vi "Draw Color Band.vi"(8 "error in (no error)":errorcluster, 9 "Range":dbl, 10 "Ideal":dbl, 11 "GaugeIndicator in":refnum<class "GaugeIndicator.lvclass">) -> (0 "error out":errorcluster, 2 "Color Band":picture, 3 "GaugeIndicator out":refnum<class "GaugeIndicator.lvclass">)   [LabVIEW 2020, in "VolatusGUIElements.lvlib" / "GaugeIndicator.lvclass"]
uses:
  GaugeIndicator.lvclass
  GaugeIndicator.lvclass/GaugeIndicator.ctl
panel:
  in  "Gauge":dbl(knob)=1600.0 scale=0.0..2500.0
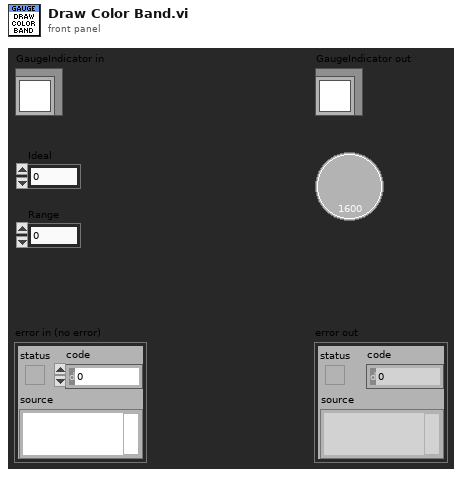
[diagram p1: front panel]
types:
  T1 = cluster{"Width":u16, "Style":enum32{"Solid", "Dash", "Dot", "DashDot", "DashDotDot"}}
  T2 = cluster{"left":i16, "top":i16, "right":i16, "bottom":i16}
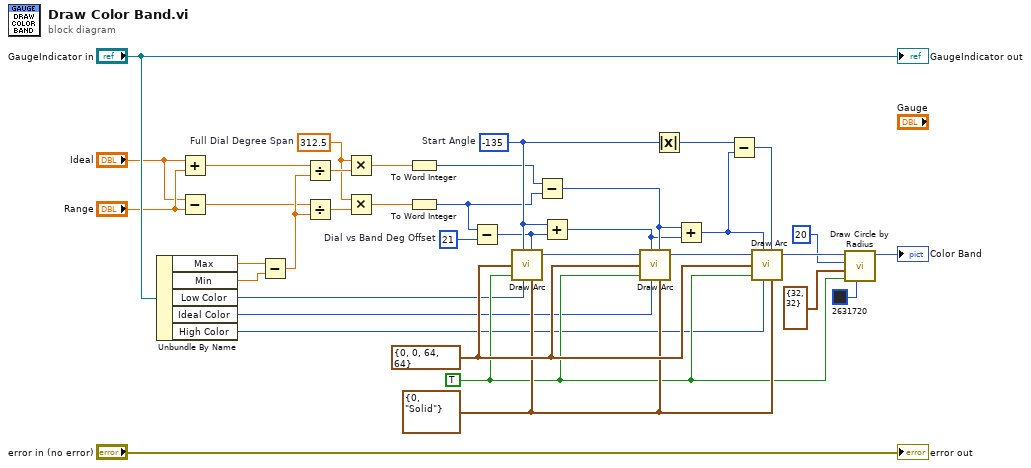
[diagram p0: block diagram]
diagram:
  w7 = i16 21  # Dial vs Band Deg Offset
  w14 = 312.5  # Full Dial Degree Span
  w10 = i16 -135  # Start Angle
  w34 = T1 {"Width"=0, "Style"=enum."Solid"} ("pen")
  w29 = TRUE ("fill?(F)")
  w35 = T2 {"left"=0, "top"=0, "right"=64, "bottom"=64} ("rect")
  n1 = Unbundle By Name("GaugeIndicator in") -> ("Max"=w22:dbl, "Min"=w21:dbl, "Low Color"=w25:u32, "Ideal Color"=w24:u32, "High Color"=w23:u32)
  n2 = Add(x="Ideal", y="Range") -> (x+y=w12:dbl)
  n3 = Subtract(x="Ideal", y="Range") -> (x-y=w8:dbl)
  n4 = Subtract(x=w22, y=w21) -> (x-y=w15:dbl)
  n5 = Divide(x=w12, y=w15) -> (x/y=w19:dbl)
  n6 = Divide(x=w8, y=w15) -> (x/y=w18:dbl)
  n7 = Multiply(x=w14, y=w19) -> (x*y=w11:dbl)
  n8 = Multiply(x=w14, y=w18) -> (x*y=w13:dbl)
  n9 = To Word Integer(number=w11) -> (16bit integer=w6:i16)
  n10 = To Word Integer(number=w13) -> (16bit integer=w3:i16)
  n11 = Subtract(x=w3, y=w7) -> (x-y=w2:i16)
  n12 = call <vilib>:"Draw Arc.vi"("start angle[degrees]"=w10, "rect"=w35, "fill?(F)"=w29, "color(black)"=w25, "arc size[degrees]"=w2, "pen"=w34) -> ("new picture"=w36:picture)  [unwired: 3 in]
  n13 = Subtract(x=w6, y=w3) -> (x-y=w5:i16)
  n14 = Add(x=w10, y=w2) -> (x+y=w4:i16)
  n15 = call <vilib>:"Draw Arc.vi"("picture"=w36, "start angle[degrees]"=w4, "rect"=w35, "fill?(F)"=w29, "color(black)"=w24, "arc size[degrees]"=w5, "pen"=w34) -> ("new picture"=w33:picture)  [unwired: 2 in]
  n16 = Absolute Value(x=w10) -> (abs(x)=w17:i16)
  n17 = Add(x=w5, y=w4) -> (x+y=w9:i16)
  n18 = Subtract(x=w17, y=w9) -> (x-y=w16:i16)
  n19 = call <vilib>:"Draw Arc.vi"("picture"=w33, "start angle[degrees]"=w9, "rect"=w35, "fill?(F)"=w29, "color(black)"=w23, "arc size[degrees]"=w16, "pen"=w34) -> ("new picture"=w32:picture)  [unwired: 2 in]
  n20 = call <vilib>:"Draw Circle by Radius.vi"("color(black)"=u32 2631720, "fill?(F)"=w29, "pixel center"=cluster{"horizontal":i16, "vertical":i16} {"horizontal"=32, "vertical"=32}, "radius"=i16 20, "picture"=w32) -> ("new picture"=→"Color Band":picture)  [unwired: 6 in]
  "error out" <- "error in (no error)"
  "GaugeIndicator out" <- "GaugeIndicator in"
